vi "三角波形.vi"(0 "sampling info":cluster{"Fs":dbl, "#s":dbl}={"Fs"=1000.0, "#s"=1000.0} caption="采样信息" {"Fs" format="%.2p"}, 5 "相位":dbl format="%.2p", 7 "偏移量":dbl format="%0.2p", 9 "频率":dbl=10.0 format="%0.2p", 11 "幅值":dbl=1.0 format="%0.2p") -> (6 "Y":dbl[](array[numeric]))   [LabVIEW 2010]
uses:
  <vilib>/measure/NI_MABase.lvlib
panel:
  in  "停止":bool
  out "dt":dbl
  out "波形图表":waveform(dbl)(graph)
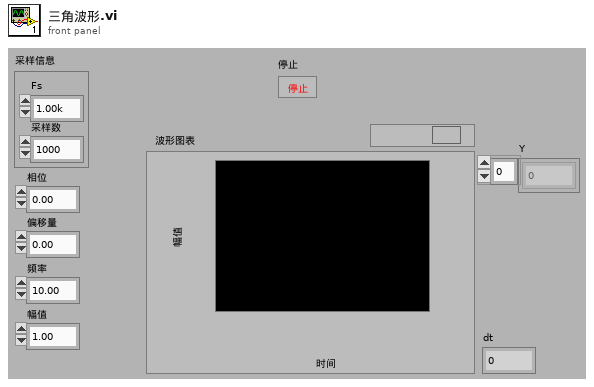
[diagram p1: front panel]
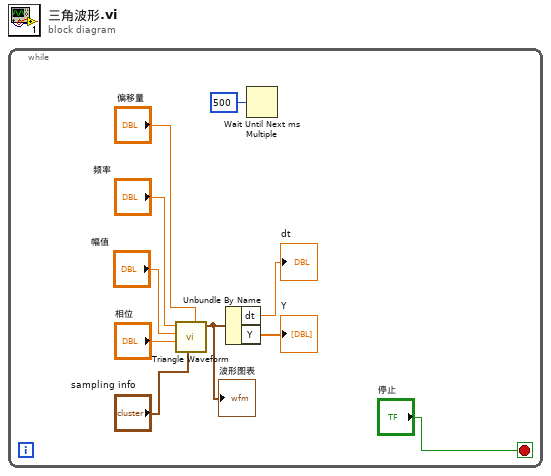
[diagram p0: block diagram]
diagram:
  n1 = while {
    stop <- "停止" stop-if-true
    n2 = call <vilib>:"Triangle Waveform.vi"("offset"="偏移量", "sampling info"="sampling info", "phase"="相位", "amplitude"="幅值", "frequency"="频率") -> ("signal out"=w5:waveform(dbl))  [unwired: 5 in, 1 out]
    "波形图表" <- w5
    n3 = Unbundle By Name(w5) -> ("dt"=→"dt":dbl, "Y"=→"Y":dbl[])
    n4 = Wait Until Next ms Multiple(millisecond multiple=u32 500 ("毫秒倍数")) -> ()  [unwired: 1 out]
  }
